vi "Create FPGA Data Node - Top.vi"(6 "LabVIEW Project to Script":path, 7 "Curent Bus Path":path, 8 "error in":errorcluster, 9 "Device Channels":i32[](array[numeric]), 10 "Bus Number":i32, 11 "Device Info":T1) -> (0 "error out":errorcluster, 3 "New Node Paths":path[](array[path]))   [LabVIEW 2014, in "SPI Engine Scripting.lvlib"]
doc: "Creates a number of IO Nodes equal to the number of channels for the current bus and adds them to a project folder and bus library."
uses:
  SPI Engine Scripting.lvlib
  State Machine/Controls/Bus Information.ctl
  State Machine/Controls/Device Information.ctl
  <vilib>/LabVIEW Icon API/API_Text.ctl
  State Machine/Controls/Pin Information.ctl
  State Machine/Controls/Values for Naming.ctl
  <vilib>/LabVIEW Icon API/LabVIEW Icon API.lvlib
panel:
  in  "New Virtual Folder":refnum<vi>
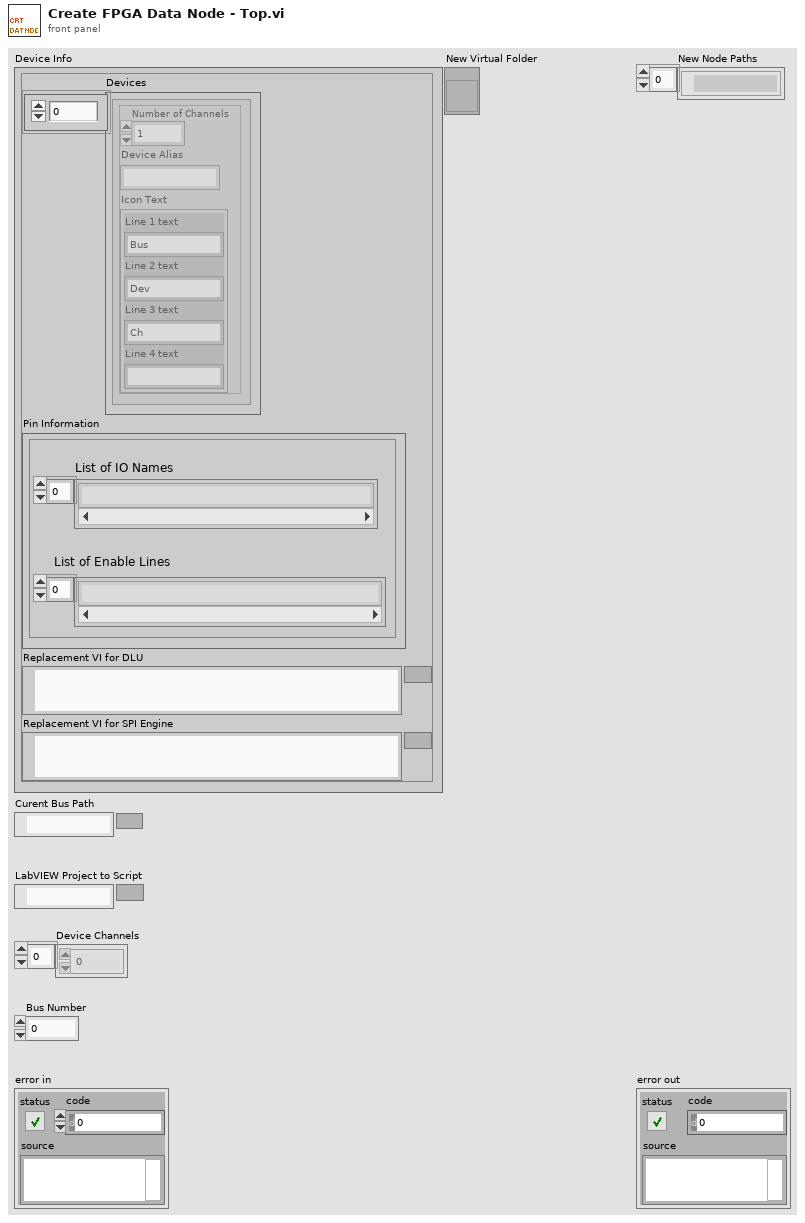
[diagram p1: front panel]
types:
  T1 = typedef "SPI Engine Scripting.lvlib/Bus Information.ctl" = cluster{"Devices":T2[], "Pin Information":T4, "Replacement VI for DLU":path, "Replacement VI for SPI Engine":path}
  T2 = typedef "Device Information.ctl" = cluster{"Number of Channels":i32, "Device Alias":string, "Icon Text":T3}
  T3 = typedef "LabVIEW Icon API.lvlib/API_Text.ctl" = cluster{"Line 1 text":string, "Line 2 text":string, "Line 3 text":string, "Line 4 text":string}
  T4 = typedef "Pin Information.ctl" = cluster{"List of IO Names":string[], "List of Enable Lines":string[]}
  T5 = typedef "SPI Engine Scripting.lvlib/Values for Naming.ctl" = cluster{"Bus Number":i32, "Device Number":i32, "Channel Number":i32}
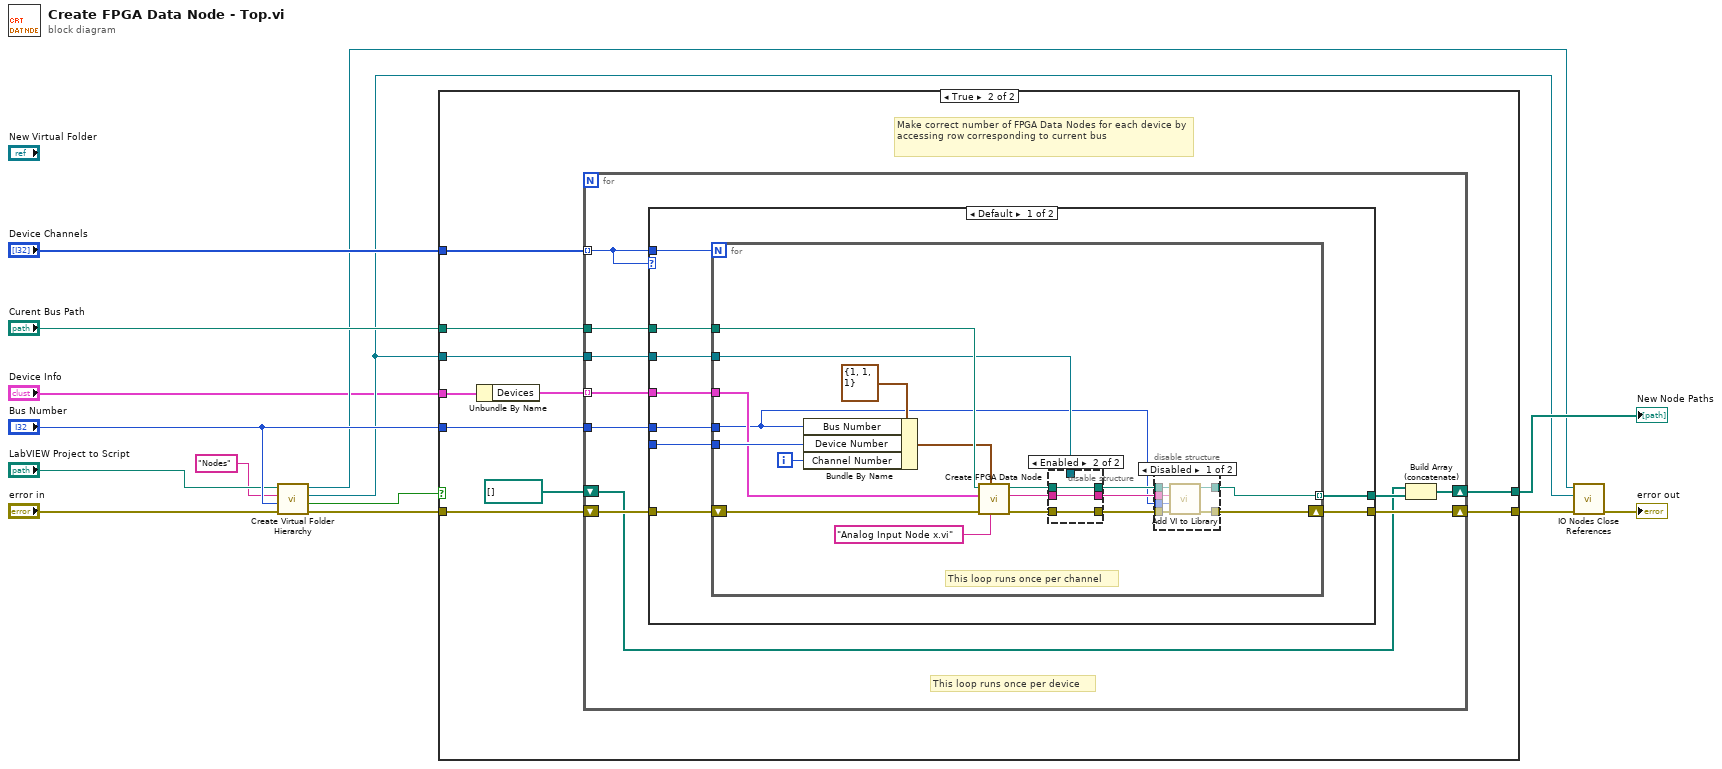
[diagram p0: block diagram]
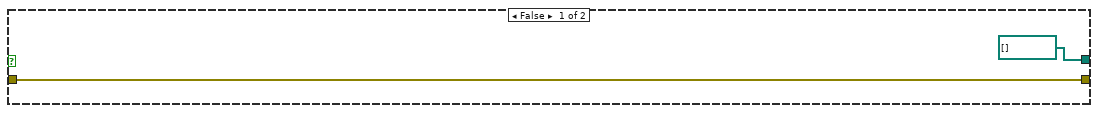
[diagram p2: hidden frame]
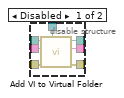
[diagram p4: hidden frame]
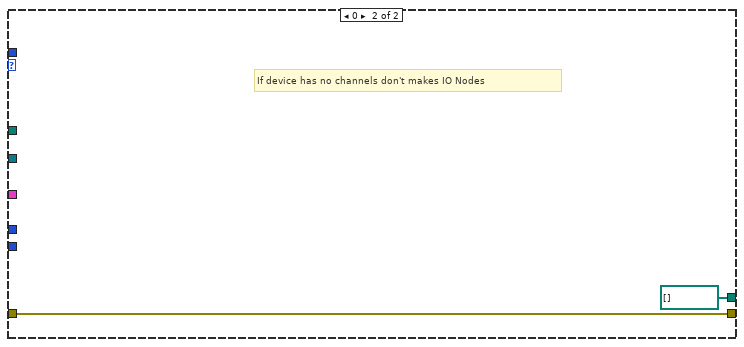
[diagram p5: hidden frame]
diagram:
  n1 = call "Create Virtual Folder Hierarchy.vi"("error in"="error in", "Bus Number"="Bus Number", "Virtual Folder Name"="Nodes", "Path to Project"="LabVIEW Project to Script") -> ("error out"=w4:errorcluster, "FPGA Target Found"=w9:bool, "New Virtual Folder"=w2:refnum<vi>, "Project:Open"=w3:refnum<vi>)  [unwired: 4 in]
  n2 = case shown="True" w9 {
    tunnel: [w15 w26] -> w13
    tunnel: "Device Channels" -> [_ w22]
    tunnel: "Bus Number" -> [_ w25]
    tunnel: "Curent Bus Path" -> [_ w24]
    tunnel: w2 -> [_ w23]
    tunnel: [path[] [] w21] -> w5
    tunnel: w4 -> [w15 w20]
    tunnel: "Device Info" -> [_ w18]
    frame False {
    }
    frame True {
      # "Make correct number of FPGA Data Nodes for each device by accessing row corresponding to current bus"
      n3 = Unbundle By Name(w18) -> ("Devices"=w17:T2[])
      n4 = for {
        shift-right: [w37] -> w26
        shift-left: w20 -> [w36]
        tunnel: w22 -> [w27] mode=indexing
        tunnel: w25 -> [w34]
        tunnel: w24 -> [w33]
        tunnel: w23 -> [w32]
        tunnel: w17 -> [w31] mode=indexing
        shift-right: [w29] -> w21
        shift-left: path[] [] -> [w28]
        i -> [w35]
        # "This loop runs once per device"
        n5 = case shown="Default" w27 {
          tunnel: [w46 w84] -> w37
          tunnel: w36 -> [w45 w84]
          tunnel: w35 -> [w44 _]
          tunnel: w27 -> [w43 _]
          tunnel: w34 -> [w42 _]
          tunnel: w33 -> [w41 _]
          tunnel: w32 -> [w40 _]
          tunnel: w31 -> [w39 _]
          tunnel: [w38 path[] []] -> w30
          frame Default {
            n6 = for {
              N: w43 -> [_]
              shift-right: [w50] -> w46
              shift-left: w45 -> [w57]
              tunnel: w44 -> [w64]
              tunnel: w42 -> [w47]
              tunnel: w41 -> [w55]
              tunnel: w40 -> [w54]
              tunnel: w39 -> [w56]
              tunnel: [w49] -> w38 mode=indexing
              i -> [w63]
              # "This loop runs once per channel"
              n7 = Bundle By Name(cluster=T5 {"Bus Number"=1, "Device Number"=1, "Channel Number"=1} ("Values for Naming"), "Bus Number"=w47, "Device Number"=w64, "Channel Number"=w63) -> (w48:T5)
              n8 = call "Create FPGA Data Node.vi"("Path to Analog Node Template"="Analog Input Node x.vi", "Values for Naming"=w48, "error in"=w57, "Device Information"=w56, "Path to IO Node"=w55) -> ("error out"=w58:errorcluster, "IO Node Name"=w59:string, "Path to new IO Node"=w60:path)  [unwired: 4 in]
              n9 = disable-structure shown="Enabled" {
                disable-tunnel: w60 -> [w79 w82]
                disable-tunnel: w59 -> [w78 w81]
                disable-tunnel: w58 -> [w77 w80]
                disable-tunnel: w54 -> [w76 _]
                disable-tunnel: [w75 w80] -> w53
                disable-tunnel: [w74 w81] -> w52
                disable-tunnel: [w73 w82] -> w51
                frame Disabled {
                  n10 = call "Add VI to Virtual Folder.vi"("Virtual Folder"=w76, "error in"=w77, "VI Name"=w78, "Path to VI"=w79) -> ("error out"=w75:errorcluster, "VI Name"=w74:string, "Path to VI"=w73:path)  [unwired: 5 in]
                }
                frame Enabled {
                }
              }
              n11 = disable-structure shown="Disabled" {
                disable-tunnel: w53 -> [w70 w72]
                disable-tunnel: w52 -> [w69 _]
                disable-tunnel: w51 -> [w68 w71]
                disable-tunnel: [w67 w72] -> w50
                disable-tunnel: [w66 w71] -> w49
                disable-tunnel: w47 -> [w65 _]
                frame Disabled {
                  n12 = call "Add VI to Library.vi"("error in"=w70, "Bus Number"=w65, "VI Name"=w69, "Path to new VI"=w68) -> ("error out"=w67:errorcluster, "Path to new IO Node"=w66:path)  [unwired: 6 in]
                }
                frame Enabled {
                }
              }
            }
          }
          frame 0 {
            # "If device has no channels don't makes IO Nodes"
          }
        }
        n13 = Build Array (concatenate)(w28, w30) -> (w29:path[])
      }
    }
  }
  "New Node Paths" <- w5
  n14 = call "IO Nodes Close References.vi"("error in (no error)"=w13, "Virtual Folder"=w2, "Project in"=w3) -> ("error out"=→"error out":errorcluster)  [unwired: 8 in]
